vi "Edit Frame.vi"(8 "error in (no error)":errorcluster, 11 "Node Ptr":u64 format="%.0x") -> (0 "error out":errorcluster)   [LabVIEW 2019, in "Diagnostics Addon System Explorer.lvlib"]
uses:
  Diagnostics Addon System Explorer.lvlib
  Types/FG.Action.ctl
  SubVIs/Signal.FG.vi
  Addon Shared/SubVIs/Constants.vi
  <vilib>/NI VeriStand/Custom Device Tools/Custom Device Utility Library/NI VeriStand - Search for Item.vi
  <vilib>/NI VeriStand/Custom Device Tools/Custom Device Utility Library/NI VeriStand - Search for Item by GUID.vi
  <vilib>/NI/NI VeriStand Advanced SysDef API/SysDef API/SysDef.Property.Set.vi
  <vilib>/NI/NI VeriStand Advanced SysDef API/_SubVIs/SysDef.Property.Set.U32.vi
  <vilib>/NI/NI VeriStand Advanced SysDef API/_SubVIs/SysDef.Property.Set.DBL.vi
  <vilib>/NI/NI VeriStand Advanced SysDef API/_SubVIs/SysDef.Property.Set.String.vi
  <vilib>/NI VeriStand/Custom Device API/NI VeriStand - Get Item Property.vi
  <vilib>/NI VeriStand/Custom Device API/Get Item Property (U32).vi
  <vilib>/NI VeriStand/Custom Device API/Get Item Property (Double).vi
  <vilib>/NI VeriStand/Custom Device API/Get Item Property (String).vi
  <vilib>/NI VeriStand/Custom Device API/NI VeriStand - Get Custom Device Channel Data.vi
  <vilib>/NI VeriStand/Custom Device API/Custom Device API.lvlib
  Addon Shared/Diagnostics Addon Shared.lvlib
  <vilib>/NI VeriStand/Custom Device Tools/Custom Device Utility Library/Custom Device Utility Library.lvlib
panel:
  in  "Tag":string
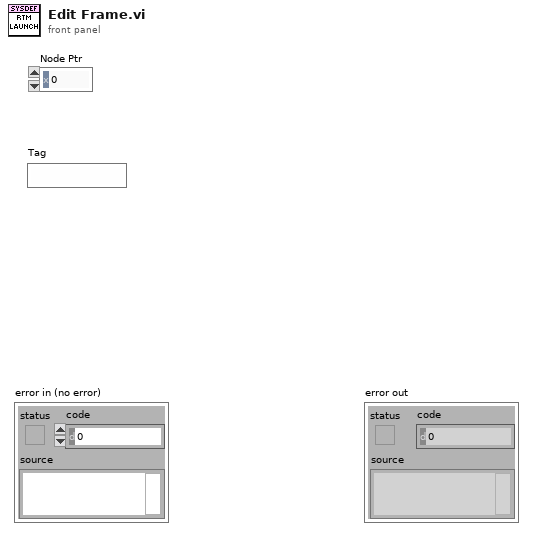
[diagram p1: front panel]
types:
  T1 = typedef "Diagnostics Addon Shared.lvlib/Signal.ctl" = cluster{"Start Bit":u32, "Length":u32, "Scaling Factor":dbl, "Scaling Offset":dbl, "Minimum":dbl, "Maximum":dbl, "Data Type":u32, "Byte Order":u32, "Default Value":dbl, "Name":string, "Units":string}
  T2 = typedef "Custom Device API.lvlib/Custom Device Item Ref.ctl" = u64
  T3 = typedef "Custom Device API.lvlib/Custom Device Item Info.ctl" = cluster{"Name":string, "Is Channel":bool, "GUID":string, "Is Waveform":bool}
  T4 = typedef "Diagnostics Addon System Explorer.lvlib/FG.Action.ctl" = enum16{"Get", "Set"}
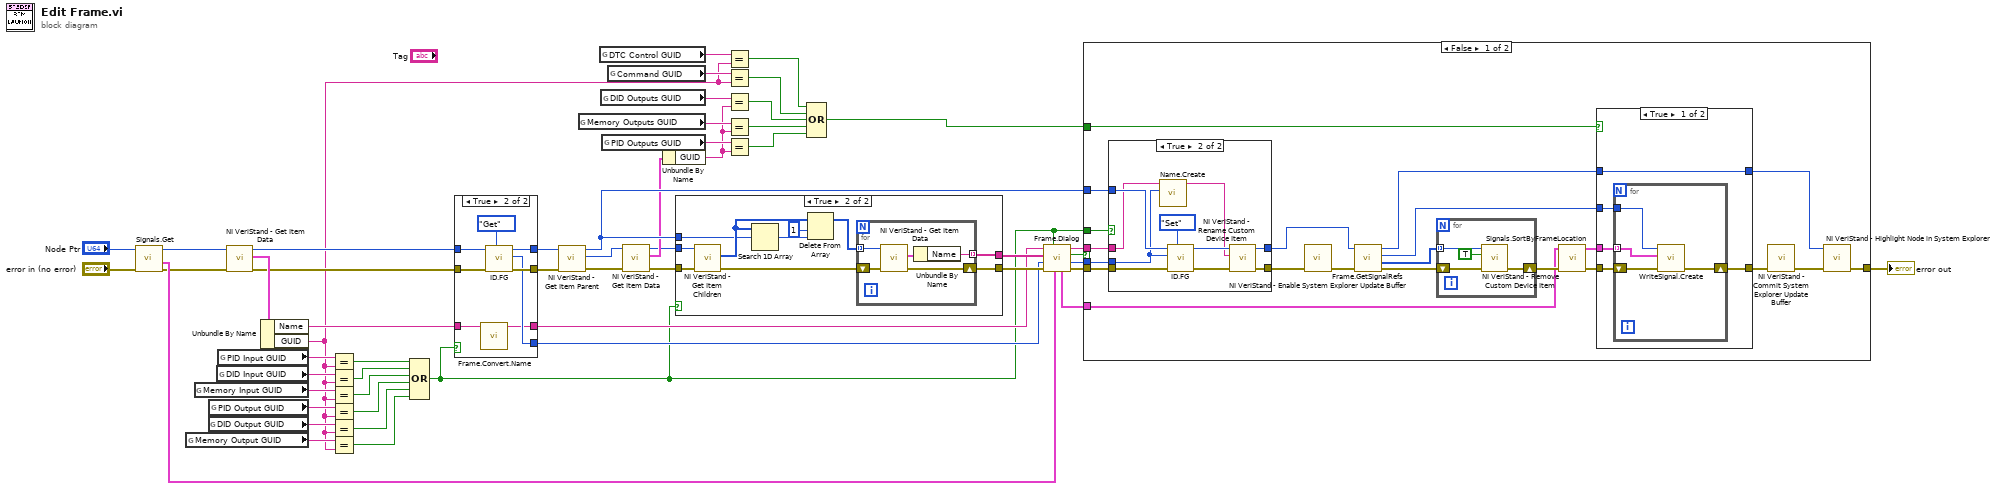
[diagram p0: block diagram]
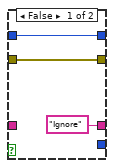
[diagram p3: hidden frame]
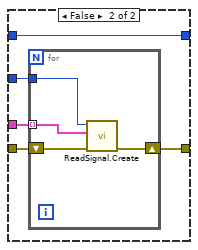
[diagram p5: hidden frame]
diagram:
  n1 = call "Signals.Get.vi"("error in (no error)"="error in (no error)", "Device Item Ref out"="Node Ptr") -> ("error out"=w34:errorcluster, "Parameters"=w36:T1[], "Item Ref out"=w35:T2)  [unwired: 6 in, 1 out]
  n2 = global read "Constants.vi" "Memory Output GUID"() -> (w7:string)
  n3 = global read "Constants.vi" "Memory Input GUID"() -> (w15:string)
  n4 = global read "Constants.vi" "DID Output GUID"() -> (w5:string)
  n5 = global read "Constants.vi" "PID Output GUID"() -> (w6:string)
  n6 = global read "Constants.vi" "DID Input GUID"() -> (w33:string)
  n7 = global read "Constants.vi" "PID Input GUID"() -> (w31:string)
  n8 = call <vilib>:"NI VeriStand - Get Item Data.vi"("error in (no error)"=w34, "Item Ref in"=w35) -> ("error out"=w29:errorcluster, "Item Info"=w32:T3, "Item Ref out"=w30:T2)  [unwired: 6 in, 1 out]
  n9 = Unbundle By Name(w32) -> ("Name"=w23:string, "GUID"=w4:string)
  n10 = Equal?(x=w31, y=w4) -> (x = y?=w28:bool)
  n11 = Equal?(x=w33, y=w4) -> (x = y?=w27:bool)
  n12 = Equal?(x=w15, y=w4) -> (x = y?=w14:bool)
  n13 = Equal?(x=w6, y=w4) -> (x = y?=w3:bool)
  n14 = Equal?(x=w5, y=w4) -> (x = y?=w2:bool)
  n15 = Equal?(x=w7, y=w4) -> (x = y?=w1:bool)
  n16 = Compound Arithmetic op=OR(w28, w27, w14, w3, w2, w1) -> (w18:bool)
  n17 = case shown="True" w18 {
    tunnel: w30 -> [w55 w59]
    tunnel: w29 -> [w56 w60]
    tunnel: [w56 w63] -> w26
    tunnel: [w55 w62] -> w25
    tunnel: [_ w61] -> w24
    tunnel: ["Ignore" ("Name") w57] -> w22
    tunnel: w23 -> [_ w58]
    frame False {
    }
    frame True {
      n18 = call "Frame.Convert.Name.vi"("VS Frame Name"=w58) -> ("Frame Name"=w57:string)  [unwired: 9 in, 1 out]
      n19 = call "ID.FG.vi"("Action"=FG.Action."Get", "error in (no error)"=w60, "Device Item Ref in"=w59) -> ("error out"=w63:errorcluster, "ID"=w61:u32, "Device Item Ref out"=w62:T2)  [unwired: 6 in]
    }
  }
  n20 = call <vilib>:"NI VeriStand - Get Item Parent.vi"("error in (no error)"=w26, "Item Ref in"=w25) -> ("error out"=w44:errorcluster, "Parent Ref"=w43:T2, "Item Ref out"=w48:T2)  [unwired: 6 in, 1 out]
  n21 = global read "Constants.vi" "Memory Outputs GUID"() -> (w16:string)
  n22 = global read "Constants.vi" "DTC Control GUID"() -> (w11:string)
  n23 = global read "Constants.vi" "DID Outputs GUID"() -> (w13:string)
  n24 = global read "Constants.vi" "PID Outputs GUID"() -> (w45:string)
  n25 = global read "Constants.vi" "Command GUID"() -> (w21:string)
  n26 = call <vilib>:"NI VeriStand - Get Item Data.vi"("error in (no error)"=w44, "Item Ref in"=w43) -> ("error out"=w41:errorcluster, "Item Info"=w46:T3, "Item Ref out"=w42:T2)  [unwired: 6 in, 1 out]
  n27 = Unbundle By Name(w46) -> ("GUID"=w12:string)
  n28 = case shown="True" w18 {
    tunnel: [w65 w70] -> w50
    tunnel: [_ w69] -> w49
    tunnel: w48 -> [_ w68]
    tunnel: w42 -> [_ w67]
    tunnel: w41 -> [w65 w66]
    frame False {
    }
    frame True {
      n29 = call <vilib>:"NI VeriStand - Get Item Children.vi"("error in (no error)"=w66, "Item Ref in"=w67) -> ("error out"=w75:errorcluster, "Child Refs"=w74:T2[])  [unwired: 6 in, 2 out]
      n30 = Search 1D Array(1D array=w74, element=w68) -> (index of element=w72:i32)  [unwired: 1 in]
      n31 = Delete From Array(array=w74, length=1, index=w72) -> (array with subset deleted=w73:T2[])  [unwired: 1 out]
      n32 = for {
        tunnel: [w78] -> w69 mode=indexing
        shift-right: [w77] -> w70
        shift-left: w75 -> [w79]
        tunnel: w73 -> [w76] mode=indexing
        n33 = call <vilib>:"NI VeriStand - Get Item Data.vi"("error in (no error)"=w79, "Item Ref in"=w76) -> ("error out"=w77:errorcluster, "Item Info"=w80:T3)  [unwired: 8 out]
        n34 = Unbundle By Name(w80) -> ("Name"=w78:string)
      }
    }
  }
  n35 = Equal?(x=w11, y=w4) -> (x = y?=w8:bool)
  n36 = Equal?(x=w21, y=w4) -> (x = y?=w10:bool)
  n37 = Equal?(x=w13, y=w12) -> (x = y?=w9:bool)
  n38 = Equal?(x=w16, y=w12) -> (x = y?=w17:bool)
  n39 = Equal?(x=w45, y=w12) -> (x = y?=w20:bool)
  n40 = Compound Arithmetic op=OR(w8, w10, w9, w17, w20) -> (w19:bool)
  n41 = call "Frame.Dialog.vi"("Signals"=w36, "Show Name&ID"=w18, "error in (no error)"=w50, "ID"=w24, "Existing PIDs"=w49, "Name"=w22) -> ("error out"=w52:errorcluster, "ID out"=w39:u16, "Cancel PID?"=w51:bool, "Name out"=w53:string, "Signals out"=w40:T1[])  [unwired: 1 in]
  n42 = case shown="False" w51 {
    tunnel: w52 -> [w97 w136]
    tunnel: w53 -> [w96 _]
    tunnel: [w101 w136] -> w47
    tunnel: w48 -> [w98 _]
    tunnel: w19 -> [w99 _]
    tunnel: w40 -> [w89 _]
    tunnel: w39 -> [w95 _]
    tunnel: w18 -> [w93 _]
    frame False {
      n43 = case shown="True" w93 {
        tunnel: w98 -> [w102 w112]
        tunnel: w97 -> [w103 w111]
        tunnel: w96 -> [_ w106]
        tunnel: w95 -> [_ w105]
        tunnel: [w102 w108] -> w85
        tunnel: [w103 w107] -> w92
        frame False {
        }
        frame True {
          n44 = call "Name.Create.vi"("PID Number"=w105, "PID Name"=w106) -> ("VS Name"=w104:string)  [unwired: 9 in]
          n45 = call "ID.FG.vi"("Action"=FG.Action."Set", "error in (no error)"=w111, "ID"=w105, "Device Item Ref in"=w112) -> ("error out"=w110:errorcluster, "Device Item Ref out"=w109:T2)  [unwired: 5 in, 1 out]
          n46 = call <vilib>:"NI VeriStand - Rename Custom Device Item.vi"("error in (no error)"=w110, "New Name"=w104, "Item Ref in"=w109) -> ("error out"=w107:errorcluster, "Item Ref out"=w108:T2)  [unwired: 1 in, 6 out]
        }
      }
      n47 = call <vilib>:"NI VeriStand - Enable System Explorer Update Buffer.vi"("error in (no error)"=w92) -> ("error out"=w87:errorcluster)  [unwired: 10 in]
      n48 = call "Frame.GetSignalRefs.vi"("error in (no error)"=w87, "Frame Item Ref in"=w85) -> ("error out"=w86:errorcluster, "Child Refs"=w84:T2[], "Signal Collection Ref out"=w83:T2, "Original Frame Ref out"=w81:T2)  [unwired: 6 in]
      n49 = for {
        tunnel: w84 -> [w114] mode=indexing
        shift-right: [w117] -> w94
        shift-left: w86 -> [w115]
        n50 = call <vilib>:"NI VeriStand - Remove Custom Device Item.vi"("error in (no error)"=w115, "Force Delete (F)"=TRUE, "Item Ref in"=w114) -> ("error out"=w117:errorcluster)  [unwired: 7 in, 1 out]
      }
      n51 = call "Signals.SortByFrameLocation.vi"("error in (no error)"=w94, "Signals in"=w89) -> ("error out"=w90:errorcluster, "Signals out"=w88:T1[])  [unwired: 8 in]
      n52 = case shown="True" w99 {
        tunnel: w83 -> [w118 w127]
        tunnel: w88 -> [w122 w131]
        tunnel: [w121 w130] -> w100
        tunnel: w90 -> [w120 w129]
        tunnel: [w119 w128] -> w82
        tunnel: w81 -> [w119 w128]
        frame True {
          n53 = for {
            shift-right: [w124] -> w121
            shift-left: w120 -> [w126]
            tunnel: w122 -> [w125] mode=indexing
            tunnel: w118 -> [w123]
            n54 = call "WriteSignal.Create.vi"("error in (no error)"=w126, "Signal Parameters"=w125, "Section Ptr"=w123) -> ("error out"=w124:errorcluster)  [unwired: 7 in, 1 out]
          }
        }
        frame False {
          n55 = for {
            shift-right: [w134] -> w130
            shift-left: w129 -> [w135]
            tunnel: w131 -> [w133] mode=indexing
            tunnel: w127 -> [w132]
            n56 = call "ReadSignal.Create.vi"("error in (no error)"=w135, "Signal Parameters"=w133, "Section Ptr"=w132) -> ("error out"=w134:errorcluster)  [unwired: 7 in, 1 out]
          }
        }
      }
      n57 = call <vilib>:"NI VeriStand - Commit System Explorer Update Buffer.vi"("error in (no error)"=w100) -> ("error out"=w91:errorcluster)  [unwired: 10 in]
      n58 = call <vilib>:"NI VeriStand - Highlight Node in System Explorer.vi"("error in (no error)"=w91, "Item Ref in"=w82) -> ("error out"=w101:errorcluster)  [unwired: 8 in, 1 out]
    }
    frame True {
    }
  }
  "error out" <- w47
